vi "Values.vi"() -> ()   [LabVIEW 2018]
panel:
  out "Power Faults":bool[](array[boolean])
  out "Temperature Faults":bool[](array[boolean])
  out "Distance Triggers":bool[](array[boolean])
  out "Avionics Battery Voltag":i32[](array[numeric])
  out "Avionics Battery Temperature":i32[](array[numeric])
  out "Avionics Battery Voltage":i32[](array[numeric])
  out "Pressure":i32
  out "Temperatures 2":i32[](array[numeric])
  out "Temperatures 1":i32[](array[numeric])
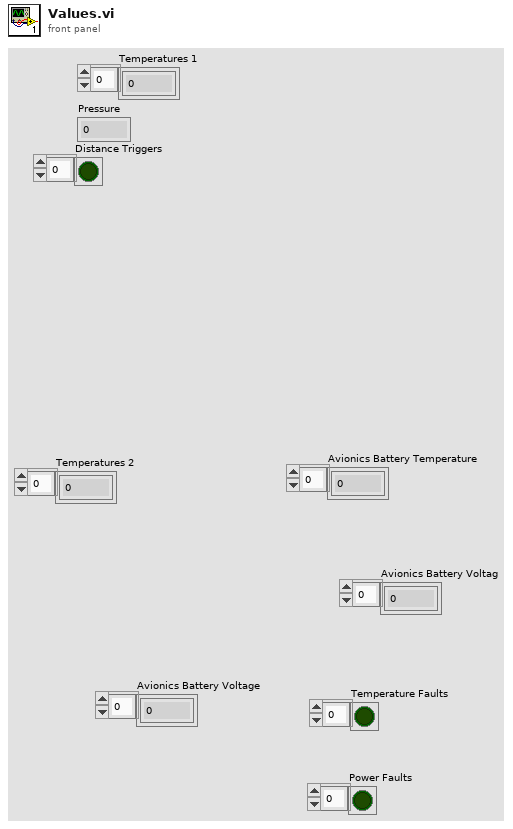
[diagram p1: front panel]
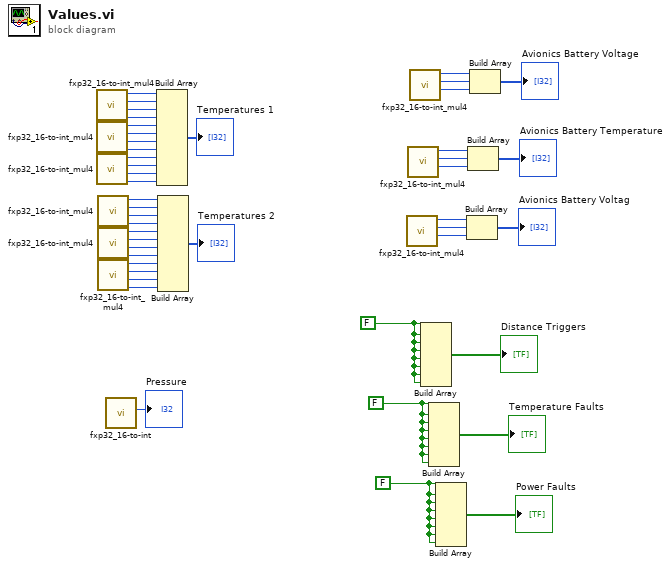
[diagram p0: block diagram]
diagram:
  w1 = FALSE
  w3 = FALSE
  w5 = FALSE
  n1 = call "fxp32_16-to-int_mul4.vi"() -> ("32bit integer 4"=w42:i32, "32bit integer 3"=w43:i32, "32bit integer 2"=w44:i32, "32bit integer 1"=w45:i32)  [unwired: 4 in]
  n2 = call "fxp32_16-to-int_mul4.vi"() -> ("32bit integer 4"=w38:i32, "32bit integer 3"=w39:i32, "32bit integer 2"=w40:i32, "32bit integer 1"=w41:i32)  [unwired: 4 in]
  n3 = call "fxp32_16-to-int_mul4.vi"() -> ("32bit integer 4"=w34:i32, "32bit integer 3"=w35:i32, "32bit integer 2"=w36:i32, "32bit integer 1"=w37:i32)  [unwired: 4 in]
  n4 = call "fxp32_16-to-int_mul4.vi"() -> ("32bit integer 4"=w29:i32, "32bit integer 3"=w30:i32, "32bit integer 2"=w31:i32, "32bit integer 1"=w32:i32)  [unwired: 4 in]
  n5 = call "fxp32_16-to-int_mul4.vi"() -> ("32bit integer 4"=w25:i32, "32bit integer 3"=w26:i32, "32bit integer 2"=w27:i32, "32bit integer 1"=w28:i32)  [unwired: 4 in]
  n6 = call "fxp32_16-to-int_mul4.vi"() -> ("32bit integer 4"=w21:i32, "32bit integer 3"=w22:i32, "32bit integer 2"=w23:i32, "32bit integer 1"=w24:i32)  [unwired: 4 in]
  n7 = call "fxp32_16-to-int.vi"() -> ("32bit integer"=→"Pressure":i32)  [unwired: 11 in]
  n8 = Build Array(w45, w44, w43, w42, w41, w40, w39, w38, w37, w36, w35, w34) -> (→"Temperatures 1":i32[])
  n9 = Build Array(w32, w31, w30, w29, w28, w27, w26, w25, w24, w23, w22, w21) -> (→"Temperatures 2":i32[])
  n10 = call "fxp32_16-to-int_mul4.vi"() -> ("32bit integer 3"=w8:i32, "32bit integer 2"=w9:i32, "32bit integer 1"=w10:i32)  [unwired: 4 in, 1 out]
  n11 = call "fxp32_16-to-int_mul4.vi"() -> ("32bit integer 3"=w12:i32, "32bit integer 2"=w13:i32, "32bit integer 1"=w14:i32)  [unwired: 4 in, 1 out]
  n12 = call "fxp32_16-to-int_mul4.vi"() -> ("32bit integer 3"=w16:i32, "32bit integer 2"=w17:i32, "32bit integer 1"=w18:i32)  [unwired: 4 in, 1 out]
  n13 = Build Array(w5, w5, w5, w5, w5, w5, w5, w5) -> (→"Distance Triggers":bool[])
  n14 = Build Array(w3, w3, w3, w3, w3, w3, w3, w3) -> (→"Temperature Faults":bool[])
  n15 = Build Array(w1, w1, w1, w1, w1, w1, w1, w1) -> (→"Power Faults":bool[])
  n16 = Build Array(w10, w9, w8) -> (→"Avionics Battery Voltag":i32[])
  n17 = Build Array(w14, w13, w12) -> (→"Avionics Battery Temperature":i32[])
  n18 = Build Array(w18, w17, w16) -> (→"Avionics Battery Voltage":i32[])
